vi "DjtgEnable.vi"(8 "Error In":errorcluster, 11 "Device Number":u32) -> (0 "Error Out":errorcluster, 3 "Device Number":u32)   [LabVIEW 2011, in "LVH-Adept.lvlib" / "DJTG.lvlib"]
doc: "This function is used to enable the default DJTG port (port 0) on the specified device. This function\nmust be called before any functions that operate on the DJTG port may be called for the specified\ndevice.s"
uses:
  DJTG.lvlib
  Private/Type Defs/Error.ctl
  <vilib>/LabVIEW Hacker/Adept/Private/Resources/djtg.dll
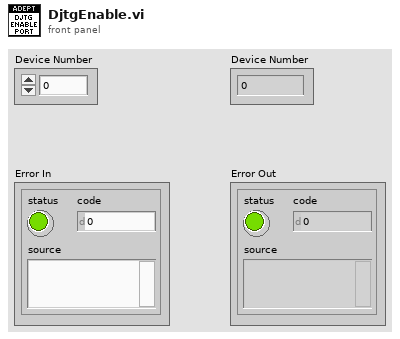
[diagram p1: front panel]
types:
  T1 = typedef "LVH-Adept.lvlib/DJTG.lvlib/Error.ctl" = enum16{"Unknown", "Enable", "PutTmsTdiBits", "GetTdoBits", "Disable", "Close", "Set Aux Reset", "Port Properties", "Get Speed", "Set Speed", "Get Port Count", "Get Batch Properties", "Enable Port", "Set Tmd Tdi Tck", "Get Tms Tdi Tdo Tck", "Put Tdi Bits", "Put Tms Bits", "Clock Tck", "Wait", "Batch", "Flash FPGA"}
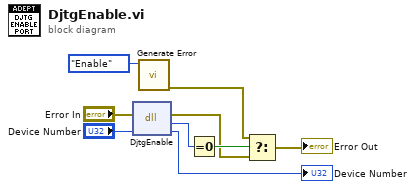
[diagram p0: block diagram]
diagram:
  n1 = dll-call lib="C:/Program Files (x86)/National Instruments/LabVIEW 2011/vi.lib/LabVIEW Hacker/Adept/Private/Resources/djtg.dll" fn="DjtgEnable"(error in="Error In", "HIF"="Device Number") -> (error out=w4:errorcluster, "Success"=w6:i32, "HIF"=→"Device Number":u32)  [unwired: 2 in, 1 out]
  n2 = call "Generate Error.vi"("DJTG Error"=Error."Enable") -> ("Error Out"=w5:errorcluster)  [unwired: 10 in]
  n3 = Equal To 0?(x=w6) -> (x = 0?=w7:bool)
  n4 = Select(t=w5, s=w7, f=w4) -> (s? t:f=→"Error Out":errorcluster)
